vi "Read Output.vi"(8 "error in (no error)":errorcluster, 10 "Channel (1: Channel 1)":i32(ring)=1 items=["Channel 1"=1, "Channel 2"=2], 11 "VISA resource name":refnum<visa-resource-name>) -> (0 "error out":errorcluster, 1 "Actual Current Level (A)":dbl format="%.2g", 2 "Actual Voltage Level (V)":dbl format="%.2g", 3 "VISA resource name out":refnum<visa-resource-name>)   [LabVIEW 2013, in "Template - DC Power.lvlib"]
doc: "Returns the actual voltage level and actual current level for a desired channel."
uses:
  <instrlib>/_Template - DC Power/Template - DC Power.lvlib
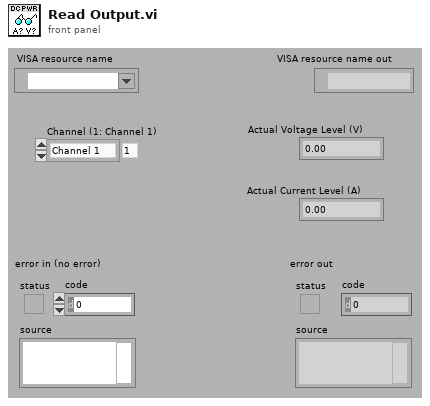
[diagram p1: front panel]
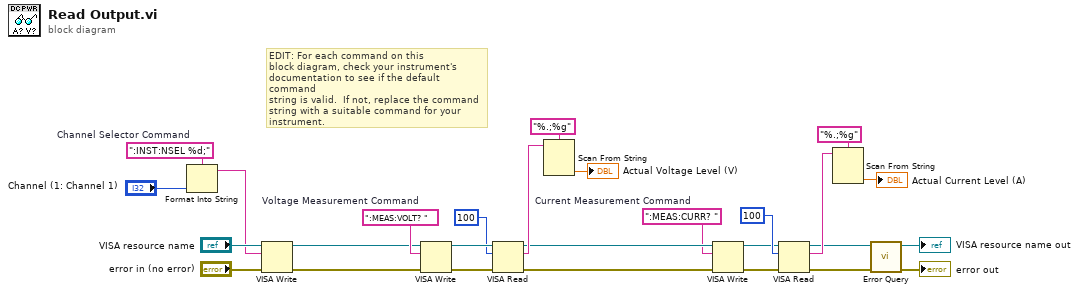
[diagram p0: block diagram]
diagram:
  w6 = ":INST:NSEL %d;"  # Channel Selector Command
  w9 = ":MEAS:CURR? "  # Current Measurement Command
  w8 = ":MEAS:VOLT? "  # Voltage Measurement Command
  # "EDIT: For each command on this\nblock diagram, check your instrument's\ndocumentation to see if the default command\nstring is valid.  If not, replace the command\nstring with a suitable command for your\ninstrument."
  n1 = Format Into String(format string=w6, "Channel (1: Channel 1)") -> (resulting string=w1:string)  [unwired: 2 in, 1 out]
  n2 = VISA Write(VISA resource name="VISA resource name", write buffer=w1, error in (no error)="error in (no error)") -> (VISA resource name out=w5:refnum<visa-resource-name>, error out=w4:errorcluster)  [unwired: 1 out]
  n3 = VISA Write(VISA resource name=w5, write buffer=w8, error in (no error)=w4) -> (VISA resource name out=w26:refnum<visa-resource-name>, error out=w27:errorcluster)  [unwired: 1 out]
  n4 = VISA Read(VISA resource name=w26, byte count=u32 100, error in (no error)=w27) -> (VISA resource name out=w10:refnum<visa-resource-name>, read buffer=w21:string, error out=w11:errorcluster)  [unwired: 1 out]
  n5 = Scan From String(format string="%.;%g", input string=w21) -> (output 1=→"Actual Voltage Level (V)":dbl)  [unwired: 3 in, 3 out]
  n6 = VISA Write(VISA resource name=w10, write buffer=w9, error in (no error)=w11) -> (VISA resource name out=w16:refnum<visa-resource-name>, error out=w15:errorcluster)  [unwired: 1 out]
  n7 = VISA Read(VISA resource name=w16, byte count=u32 100, error in (no error)=w15) -> (VISA resource name out=w13:refnum<visa-resource-name>, read buffer=w18:string, error out=w12:errorcluster)  [unwired: 1 out]
  n8 = Scan From String(format string="%.;%g", input string=w18) -> (output 1=→"Actual Current Level (A)":dbl)  [unwired: 3 in, 3 out]
  n9 = call <instrlib>:"Error Query.vi"("error in (no error)"=w12, "VISA resource name"=w13) -> ("error out"=→"error out":errorcluster, "VISA resource name out"=→"VISA resource name out":refnum<visa-resource-name>)  [unwired: 6 in, 2 out]
